vi "PDF Protokoll EPA1065_376 Chiller.vi"(8 "error in (no error)":errorcluster caption="Fehler (Eingang, kein Fehler)") -> (0 "error out":errorcluster caption="Fehler (Ausgang)")   [LabVIEW 2020, in "EPA 1065.lvlib" / "Chiller NO2 1065-376.lvlib"]
uses:
  Chiller NO2 1065-376.lvlib
  T90 1065-308/Ergebnis.ctl
  Seiten/FT-IR/FGV FT-IR Aktionen.ctl
  Seiten/System Einstellungen V2/Aktioen FGV System Konstanten.ctl
  Aktion FGV Chiller Test.ctl
  <vilib>/Utility/miscctls.llb/LVPrintingMarginsTypeDef.ctl
  Allgemein/allgemeine Sub-VIs.lvlib
  Seiten/FT-IR/FT-IR.lvlib
  Seiten/System Einstellungen V2/System Einstellungen V2.lvlib
  T90 1065-308/T90 Test 1065-308.lvlib
panel:
  out "H2O":string caption="%"
  out "xNOxmeas":string caption="ppm"
  out "Ergebnis 1":T1
  out "xNOxmeas_dry":string caption="ppm"
  out "xNOxRef":string caption="ppm"
  out "Expiry Date":string caption="Expiry Date:"
  out "Versa Serial number:":string caption="Serial number:"
  out "Anlage:":string caption="Measuring Device:"
  out "Methode (Recipe):":string
  out "Date & Time:":string
  out "Accuracy:":string
  out "Gas Bottle Nr.:":string
  out "Ergebnis:":string caption="Result:"
  out "Konzentration:":string caption="Setpoint:"
  out "Komponente:":string caption="Component:"
  out "Bearbeiter:":string caption="Operator:"
  out "Serial number:":string
  out "Messgerät:":string caption="Analyzer:"
  # "Chiller Test EPA § 1065.376"
  # "xNOxmeas_dry ="
  # "/"
  # "(1-"
  # "/ 100)"
  # "x 0.95"
  # "<"
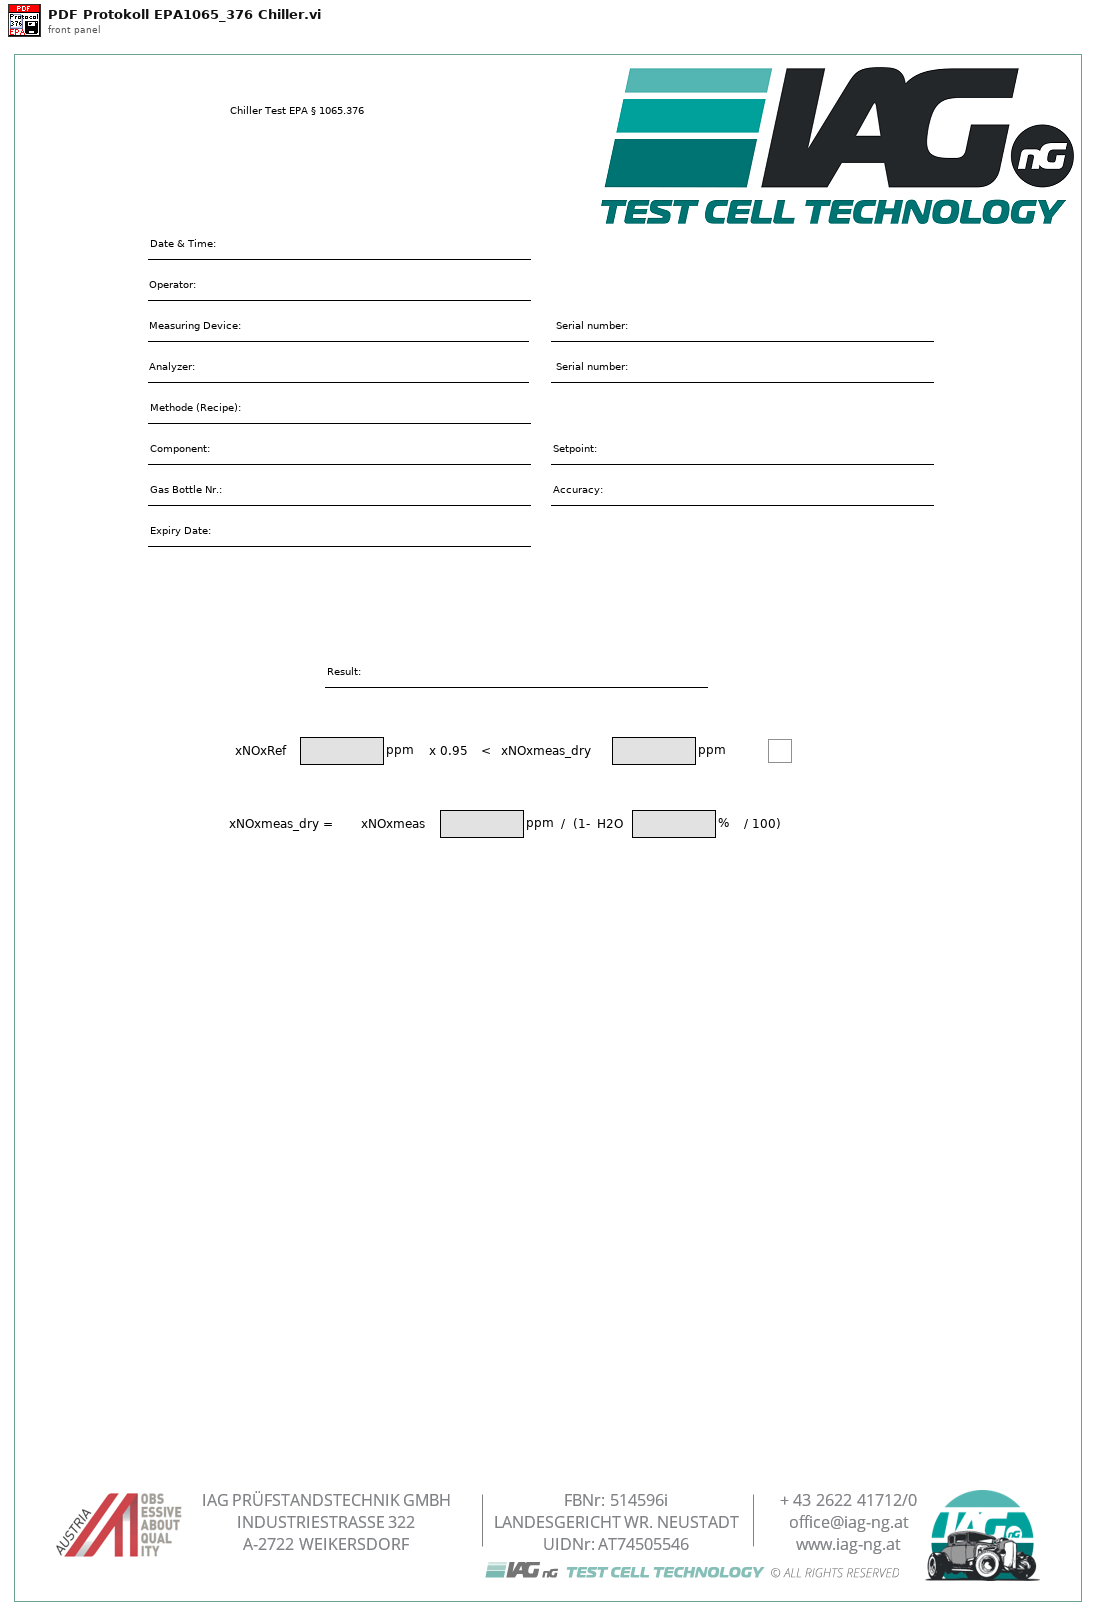
[diagram p1: front panel]
types:
  T1 = typedef "EPA 1065.lvlib/T90 Test 1065-308.lvlib/Ergebnis.ctl" = bool
  T2 = typedef "EPA 1065.lvlib/Chiller NO2 1065-376.lvlib/Aktion FGV Chiller Test.ctl" = enum16{"lesen", "Konfig Daten", "Messdaten", "Resultat", "Daten löschen", "PDF einstellen", "laden", "speichern"}
  T3 = typedef "System Einstellungen V2.lvlib/Aktioen FGV System Konstanten.ctl" = enum16{"lesen", "laden", "speichern", "Sprache"}
  T4 = typedef "FT-IR.lvlib/FGV FT-IR Aktionen.ctl" = enum16{"lesen", "NOG setzen", "NOS setzen", "Initialisieren", "speichern", "ALLES setzen", "FT-IR Spektrum loggen", "Komm Stoppen", "Spektrum LogKonfig"}
  T5 = enum32{"Portrait", "Landscape", "Rotated Portrait", "Rotated Landscape"}
  T6 = typedef "LVPrintingMarginsTypeDef.ctl" = cluster{"Top":sgl, "Left":sgl, "Bottom":sgl, "Right":sgl, "Measurement System":enum8{"Inches", "cm"}}
  T7 = typedef "EPA 1065.lvlib/Chiller NO2 1065-376.lvlib/Chiller Konfig Daten.ctl" = cluster{"Bearbeiter:":string, "Gasflaschen Nr.:":string, "Accuracy":dbl, "Sollwert":dbl, "Messgerät:":string, "Seriennummer:":string, "Pfad:":path, "Textname:":string, "Einheit":string, "Expiry Date":timestamp, "Water Concentration:":dbl, "Componente:":string}
  T8 = cluster{"Modell":string, "ProjektNummer":string, "Software Version":string, "Seriennummer":string}
  T9 = typedef "EPA 1065.lvlib/Chiller NO2 1065-376.lvlib/Messdaten.ctl" = cluster{"xNOxRef":dbl, "xNOxmeas":dbl, "H2O":dbl, "xNOx_dry":dbl, "Bestanden":bool}
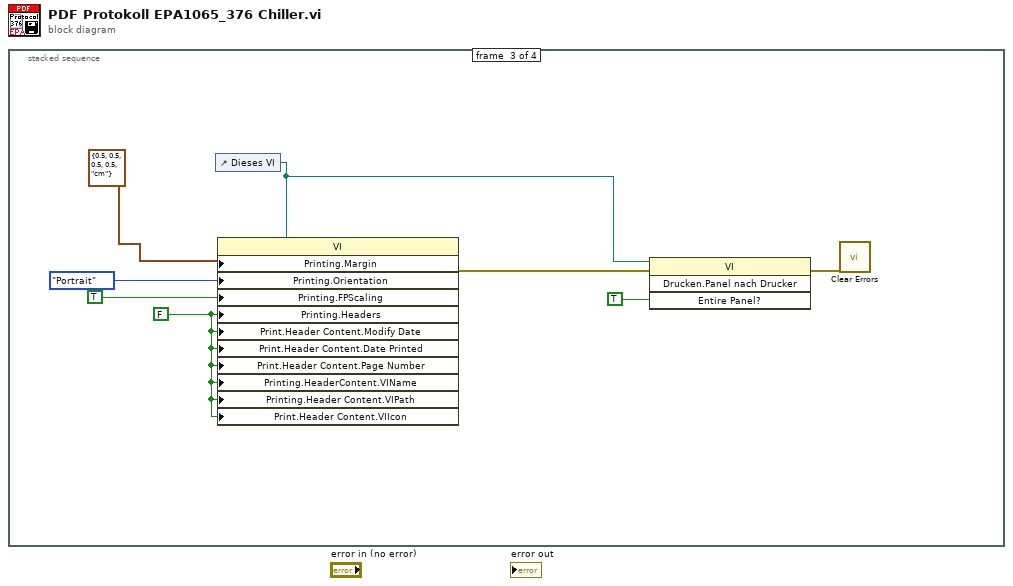
[diagram p0: block diagram]
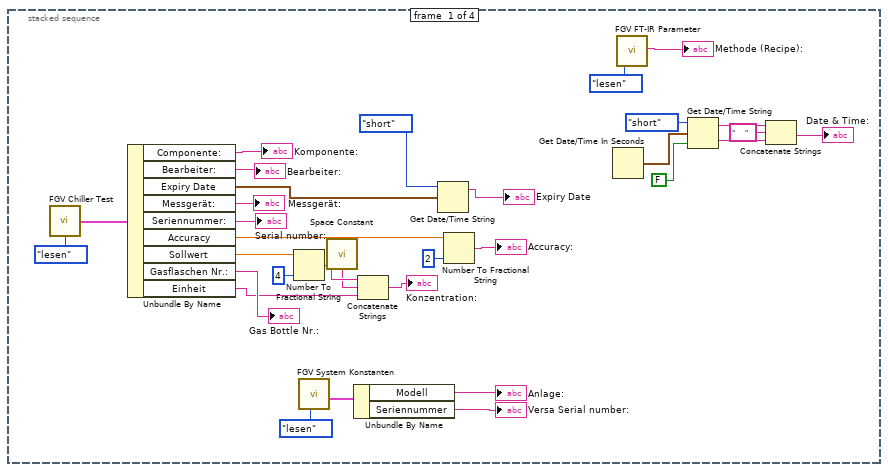
[diagram p2: hidden frame]
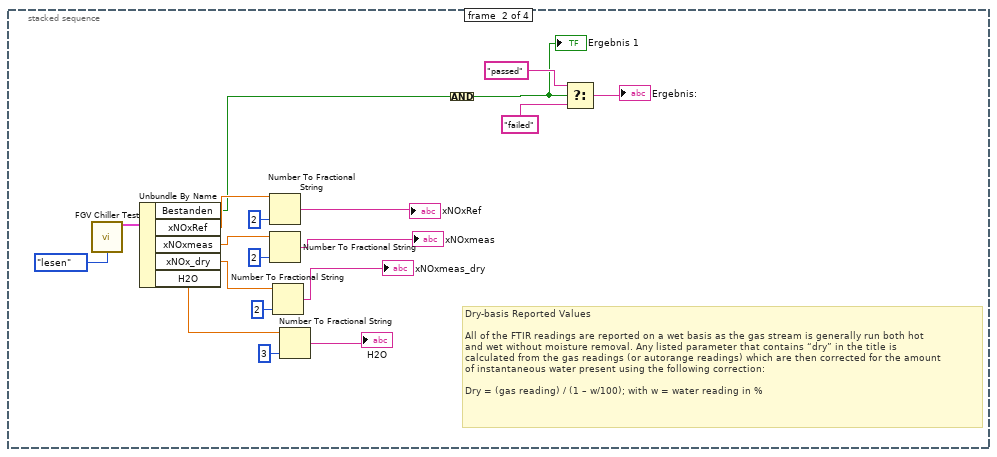
[diagram p3: hidden frame]
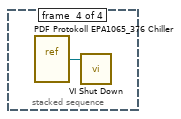
[diagram p4: hidden frame]
diagram:
  n1 = stacked-sequence {
    frame #0 {
      n2 = call "FGV Chiller Test.vi"("Aktion"=Aktion_FGV_Chiller_Test."lesen") -> ("Chiller Konfig Daten"=w6:T7)  [unwired: 11 in, 3 out]
      n3 = Unbundle By Name(w6) -> ("Componente:"=→"Komponente:":string, "Bearbeiter:"=→"Bearbeiter:":string, "Expiry Date"=w4:timestamp, "Messgerät:"=→"Messgerät:":string, "Seriennummer:"=→"Serial number:":string, "Accuracy"=w20:dbl, "Sollwert"=w16:dbl, "Gasflaschen Nr.:"=→"Gas Bottle Nr.:":string, "Einheit"=w11:string)
      n4 = Number To Fractional String(number=w16, precision (6)=i16 4 ("Genauigkeit (6)")) -> (F-format string=w14:string)  [unwired: 2 in]
      n5 = call "FGV System Konstanten.vi"("Aktionen"=Aktioen_FGV_System_Konstanten."lesen") -> ("Cluster out"=w9:T8)  [unwired: 6 in, 4 out]
      n6 = call <vilib>:"Space Constant.vi"() -> ("String"=w12:string)
      n7 = Unbundle By Name(w9) -> ("Modell"=→"Anlage:":string, "Seriennummer"=→"Versa Serial number:":string)
      n8 = Concatenate Strings(w14, w12, w11) -> (→"Konzentration:":string)
      n9 = Get Date/Time String(date format (0)=enum16{"short", "long", "abbreviated"}."short" ("Datumsformat (0)"), seconds (now)=w4) -> (date string=→"Expiry Date":string)  [unwired: 1 in, 1 out]
      n10 = Number To Fractional String(number=w20, precision (6)=i16 2 ("Genauigkeit (6)")) -> (F-format string=→"Accuracy:":string)  [unwired: 2 in]
      n11 = Get Date/Time In Seconds() -> (seconds since 1Jan1904=w32:timestamp)
      n12 = call "FGV FT-IR Parameter.vi"("Aktion"=FGV_FT-IR_Aktionen."lesen") -> ("Current Recipe"=→"Methode (Recipe):":string)  [unwired: 11 in, 7 out]
      n13 = Get Date/Time String(date format (0)=enum16{"short", "long", "abbreviated"}."short" ("Datumsformat (0)"), seconds (now)=w32, want seconds? (F)=FALSE ("Angabe von Sekunden? (F)")) -> (date string=w31:string, time string=w30:string)
      n14 = Concatenate Strings(w31, "     " ("String"), w30) -> (→"Date & Time:":string)
    }
    frame #1 {
      # "Dry-basis Reported Values\n\nAll of the FTIR readings are reported on a wet basis as the gas stream is generally run both hot\nand wet without moisture removal. Any listed parameter that contains “dry” in the title is\ncalculated from the gas readings (or autorange readings) which are then corrected for the amount\nof instantaneous water present using the following correction:\n\nDry = (gas reading) / (1 – w/100); with w = water reading in %"
      n15 = call "FGV Chiller Test.vi"("Aktion"=Aktion_FGV_Chiller_Test."lesen") -> ("Daten"=w42:T9)  [unwired: 11 in, 3 out]
      n16 = Unbundle By Name(w42) -> ("Bestanden"=w36:bool, "xNOxRef"=w41:dbl, "xNOxmeas"=w40:dbl, "xNOx_dry"=w38:dbl, "H2O"=w33:dbl)
      n17 = Number To Fractional String(number=w41, precision (6)=i16 2 ("Genauigkeit (6)")) -> (F-format string=→"xNOxRef":string)  [unwired: 2 in]
      n18 = Number To Fractional String(number=w40, precision (6)=i16 2 ("Genauigkeit (6)")) -> (F-format string=→"xNOxmeas":string)  [unwired: 2 in]
      n19 = Number To Fractional String(number=w38, precision (6)=i16 2 ("Genauigkeit (6)")) -> (F-format string=→"xNOxmeas_dry":string)  [unwired: 2 in]
      n20 = Number To Fractional String(number=w33, precision (6)=i16 3 ("Genauigkeit (6)")) -> (F-format string=→"H2O":string)  [unwired: 2 in]
      n21 = Compound Arithmetic op=AND ("Mehrfacharithmetik")(w36) -> (w35:bool)
      "Ergebnis 1" <- w35
      n22 = Select(t="passed", s=w35, f="failed") -> (s? t:f=→"Ergebnis:":string)
    }
    frame #2 {
      w55 = FALSE ("Drucken:Kopfzeilen?")
      n23 = control-ref of="Dieses VI"() -> (w52:refnum<vi>)
      n24 = property class="VI"(reference=w52, "Printing.Margin"=T6 {"Top"=0.5, "Left"=0.5, "Bottom"=0.5, "Right"=0.5, "Measurement System"=enum."cm"} ("Drucken:Ränder"), "Printing.Orientation"=T5."Portrait" ("Drucken:Seitenausrichtung"), "Printing.FPScaling"=TRUE ("Drucken:Frontpanel-Skalierung?"), "Printing.Headers"=w55, "Print.Header Content.Modify Date"=w55, "Print.Header Content.Date Printed"=w55, "Print.Header Content.Page Number"=w55, "Printing.HeaderContent.VIName"=w55, "Printing.Header Content.VIPath"=w55, "Print.Header Content.VIIcon"=w55) -> (error out=w59:errorcluster)  [unwired: 1 in, 1 out]
      n25 = invoke class="VI" method="Drucken.Panel nach Drucker"(reference=w52, error in=w59, "Entire Panel?"=TRUE ("Abschnittskopfzeilen?")) -> (error out=w53:errorcluster)  [unwired: 1 in, 3 out]
      n26 = call <vilib>:"Clear Errors.vi"("error in (no error)"=w53) -> ()  [unwired: 5 in, 2 out]
    }
    frame #3 {
      n27 = vi-ref "PDF Protokoll EPA1065_376 Chiller.vi"() -> (w60:refnum<vi>)
      n28 = call "VI Shut Down.vi"("VI Referenz"=w60) -> ()  [unwired: 11 in]
    }
  }
